vi "Sets and Query the Function on 2nd Display.vi"(5 "Enable to Query":bool=TRUE, 7 "Enable to Sets":bool=TRUE, 8 "error in":errorcluster, 10 "Function":u8(ring) items=["VOLT:DC", "VOLT:AC", "CURR:DC", "CURR:AC", "RES", "FREQ", "PER", "NON"], 11 "VISA resource name":refnum<visa-resource-name>) -> (0 "error out":errorcluster, 2 "Return the Function":string, 3 "VISA resource name out":refnum<visa-resource-name>)   [LabVIEW 2011, in "DMM4.lvlib"]
uses:
  <instrlib>/DMM4/DMM4.lvlib
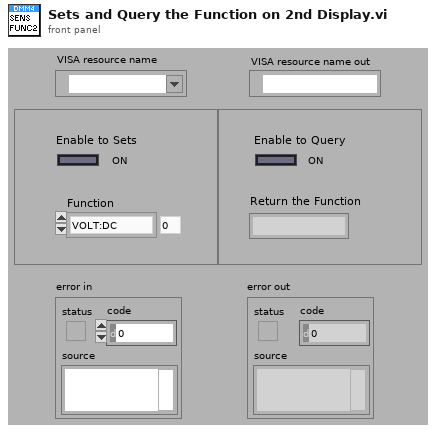
[diagram p1: front panel]
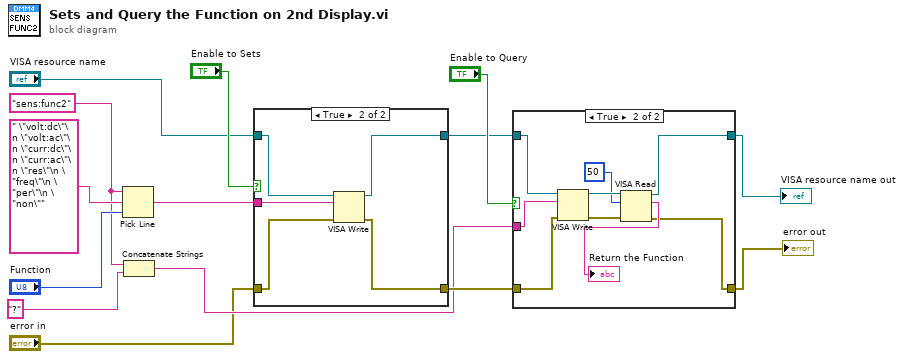
[diagram p0: block diagram]
diagram:
  w10 = "sens:func2"
  n1 = Pick Line(string ("")=w10, multi-line string=" \"volt:dc\"\n \"volt:ac\"\n \"curr:dc\"\n \"curr:ac\"\n \"res\"\n \"freq\"\n \"per\"\n \"non\"", line index="Function") -> (output string=w9:string)
  n2 = Concatenate Strings(w10, "?") -> (w4:string)
  n3 = case shown="True" "Enable to Sets" {
    tunnel: w9 -> [_ w21]
    tunnel: "VISA resource name" -> [w16 w20]
    tunnel: "error in" -> [w15 w19]
    tunnel: [w16 w18] -> w6
    tunnel: [w15 w17] -> w5
    frame False {
    }
    frame True {
      n4 = VISA Write(VISA resource name=w20, write buffer=w21, error in (no error)=w19) -> (VISA resource name out=w18:refnum<visa-resource-name>, error out=w17:errorcluster)  [unwired: 1 out]
    }
  }
  n5 = case shown="True" "Enable to Query" {
    tunnel: w6 -> [w23 w31]
    tunnel: w5 -> [w22 w30]
    tunnel: w4 -> [_ w32]
    tunnel: [w23 w25] -> w3
    tunnel: [w22 w24] -> w2
    frame False {
    }
    frame True {
      n6 = VISA Write(VISA resource name=w31, write buffer=w32, error in (no error)=w30) -> (VISA resource name out=w29:refnum<visa-resource-name>, error out=w28:errorcluster)  [unwired: 1 out]
      n7 = VISA Read(VISA resource name=w29, byte count=u32 50, error in (no error)=w28) -> (VISA resource name out=w25:refnum<visa-resource-name>, read buffer=→"Return the Function":string, error out=w24:errorcluster)  [unwired: 1 out]
    }
  }
  "VISA resource name out" <- w3
  "error out" <- w2
